vi "Save to File.vi"(8 "error in (no error)":errorcluster, 10 "Single Channel?":bool, 11 "File Control":T1) -> (0 "error out":errorcluster)   [LabVIEW 2017]
uses:
  Controls/File Controls.ctl
  <vilib>/Waveform/WDTFileIO.llb/Read Waveform from File.vi
  <vilib>/Utility/file.llb/Write Delimited Spreadsheet (DBL).vi
panel:
  out "Dev2 + Trigger Signals":dbl[][](array[numeric])
  out "Dev1 Signals":dbl[][](array[numeric])
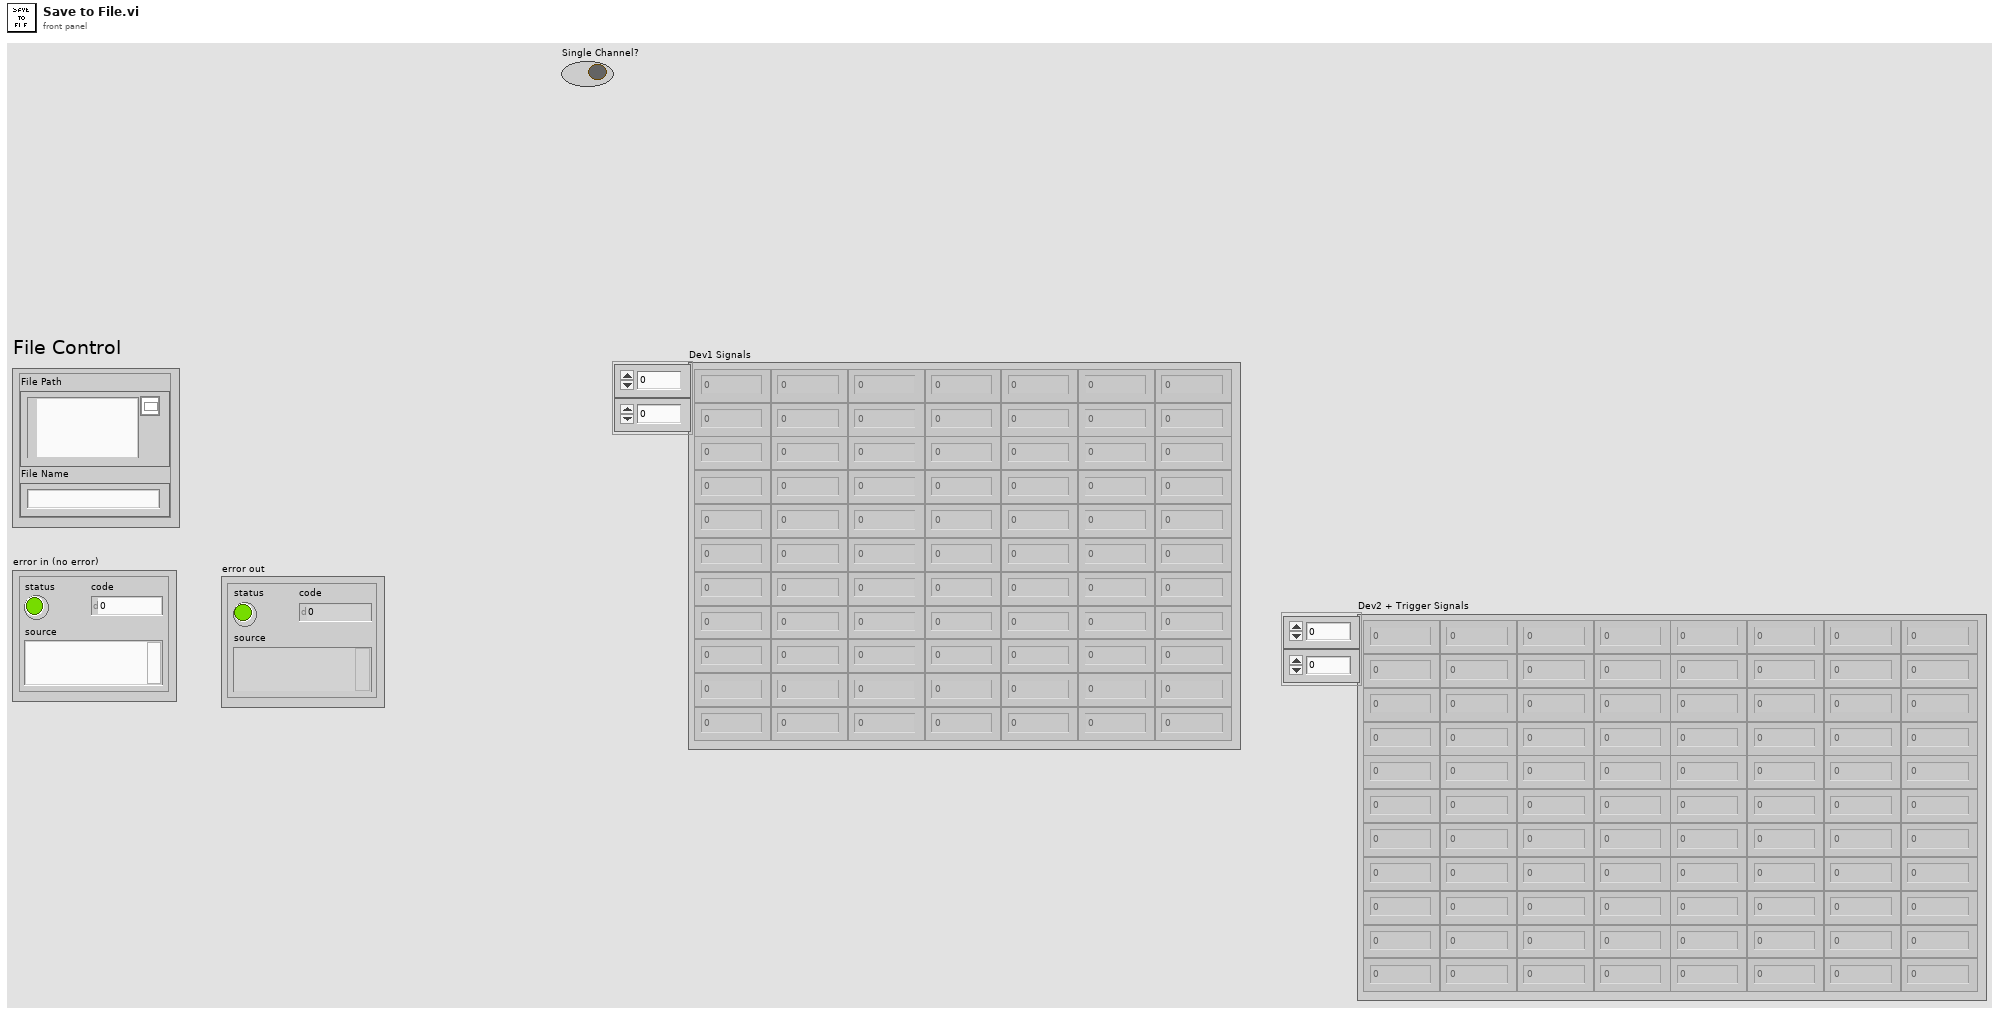
[diagram p1: front panel]
types:
  T1 = typedef "File Controls.ctl" = cluster{"File Path":path, "File Name":string}
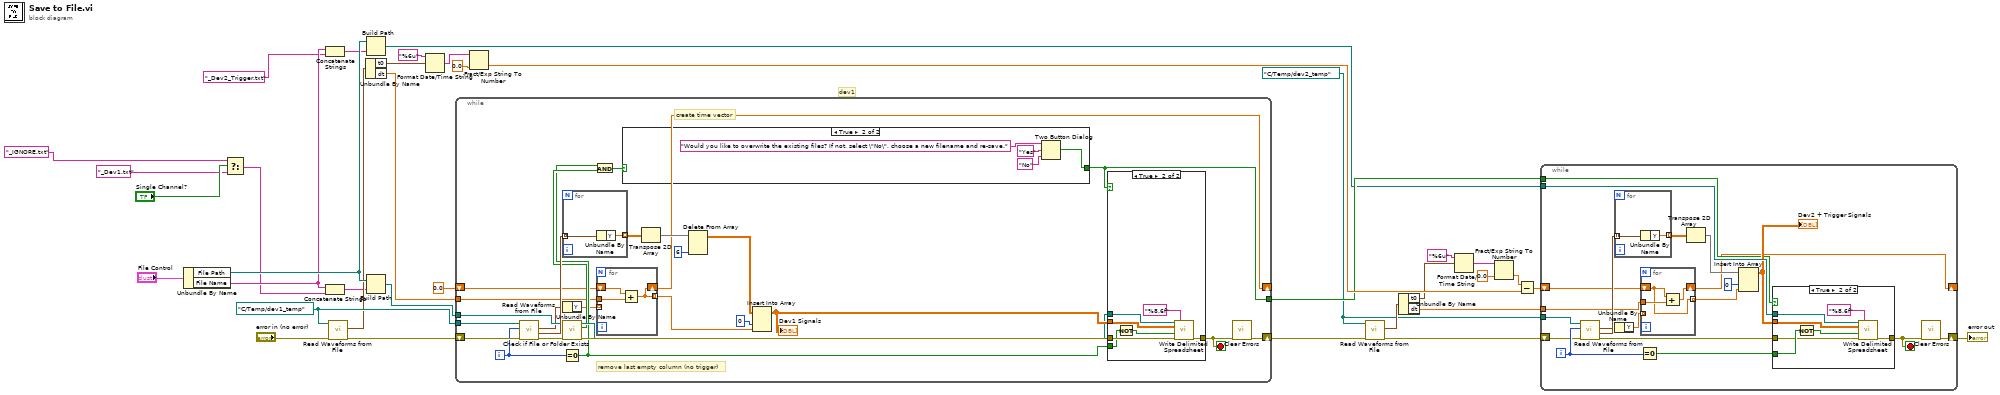
[diagram p0: block diagram]
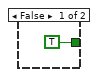
[diagram p3: hidden frame]
diagram:
  w30 = path "C:/Temp/dev1_temp" ("file path (dialog if empty)")
  w13 = path "C:/Temp/dev2_temp" ("file path (dialog if empty)")
  # "dev1"
  n1 = Unbundle By Name("File Control") -> ("File Path"=w35:path, "File Name"=w34:string)
  n2 = Select(t="_IGNORE.txt" ("string"), s="Single Channel?", f="_Dev1.txt" ("string")) -> (s? t:f=w5:string)
  n3 = Concatenate Strings(w34, "_Dev2_Trigger.txt" ("string")) -> (w33:string)
  n4 = Concatenate Strings(w34, w5) -> (w12:string)
  n5 = call-poly <vilib>:"Read Waveforms from File.vi"("error in (no error)"="error in (no error)", "file path (dialog if empty)"=w30) -> ("error out"=w8:errorcluster, "first waveform in record"=w21:waveform(dbl))  [unwired: 4 in, 2 out]
  n6 = Unbundle By Name(w21) -> ("t0"=w20:timestamp, "dt"=w17:dbl)
  n7 = Build Path(base path=w35, name or relative path=w33) -> (appended path=w10:path)
  n8 = Build Path(base path=w35, name or relative path=w12) -> (appended path=w11:path)
  n9 = Format Date/Time String(time format string (%c)="%6u", seconds (now)=w20) -> (date/time string=w26:string)  [unwired: 1 in]
  n10 = while {
    tunnel: w30 -> [w62]
    shift-right: [w51] -> w7
    shift-left: w8 -> [w61]
    shift-right: [w38] -> _
    shift-left: 0.0 -> [w40]
    tunnel: w17 -> [w41]
    tunnel: [w46] -> w16
    tunnel: w11 -> [w44]
    i -> [w48]
    stop <- w50 stop-if-true
    # "create time vector"
    # "remove last empty column (no trigger)"
    n11 = call-poly <vilib>:"Read Waveforms from File.vi"("error in (no error)"=w61, "offset (records:0)"=w48, "file path (dialog if empty)"=w62) -> ("error out"=w45:errorcluster, "all waveforms in record"=w60:waveform(dbl)[], "first waveform in record"=w43:waveform(dbl))  [unwired: 3 in, 1 out]
    n12 = for {
      tunnel: w60 -> [w80] mode=indexing
      tunnel: [w79] -> w59 mode=indexing
      n13 = Unbundle By Name(w80) -> ("Y"=w79:dbl[])
    }
    n14 = Unbundle By Name(w43) -> ("Y"=w42:dbl[])
    n15 = call <vilib>:"Check if File or Folder Exists.vi"("error in (no error)"=w45, "path"=w44) -> ("error out"=w54:errorcluster, "file or folder exists?"=w52:bool, "dup path"=w53:path)  [unwired: 7 in]
    n16 = Equal To 0?(x=w48) -> (x = 0?=w47:bool)
    n17 = And(x=w47, y=w52) -> (x .and. y?=w49:bool)
    n18 = for {
      tunnel: w42 -> [_] mode=indexing
      tunnel: w41 -> [w65]
      shift-right: [w63] -> w38
      shift-left: w40 -> [w64]
      tunnel: [w63] -> w39 mode=indexing
      n19 = Add(x=w64, y=w65) -> (x+y=w63:dbl)
    }
    n20 = case shown="True" w49 {
      tunnel: [TRUE ("T button?") w70] -> w46
      frame False {
      }
      frame True {
        n21 = Two Button Dialog(message="Would you like to overwrite the existing files? If not, select \"No\", choose a new filename and re-save.", 1:"No" ("F button name (\"Cancel\")"), 2:"Yes" ("T button name (\"OK\")")) -> (T button?=w70:bool)
      }
    }
    n22 = Transpose 2D Array(2D array=w59) -> (transposed array=w58:dbl[][])
    n23 = Delete From Array(array=w58, index (col)=6 ("disabled index (col)")) -> (array with subset deleted=w57:dbl[][])  [unwired: 2 in, 1 out]
    n24 = Insert Into Array(array=w57, index (col)=0 ("disabled index (col)"), new element=w39) -> (w55:dbl[][])  [unwired: 1 in]
    "Dev1 Signals" <- w55
    n25 = case shown="True" w46 {
      tunnel: [w71 w72] -> w50
      tunnel: w55 -> [_ w78]
      tunnel: w53 -> [_ w77]
      tunnel: w54 -> [w71 w76]
      tunnel: w47 -> [_ w74]
      frame False {
      }
      frame True {
        n26 = Not(x=w74) -> (.not. x?=w73:bool)
        n27 = call-poly <vilib>:"Write Delimited Spreadsheet.vi"("file path (dialog if empty)"=w77, "format (%.3f)"="%8.6f", "2D data"=w78, "append to file? (new file:F)"=w73, "error in (no error)"=w76) -> ("error out"=w72:errorcluster)  [unwired: 9 in, 1 out]
      }
    }
    n28 = call <vilib>:"Clear Errors.vi"("error in (no error)"=w50) -> ("error out"=w51:errorcluster)  [unwired: 5 in, 1 out]
  }
  n29 = Fract/Exp String To Number(string=w26, default (0 dbl)=0.0 ("default (0 DBL)")) -> (number=w28:dbl)  [unwired: 2 in, 1 out]
  n30 = call-poly <vilib>:"Read Waveforms from File.vi"("error in (no error)"=w7, "file path (dialog if empty)"=w13) -> ("error out"=w6:errorcluster, "first waveform in record"=w18:waveform(dbl))  [unwired: 4 in, 2 out]
  n31 = Unbundle By Name(w18) -> ("t0"=w19:timestamp, "dt"=w9:dbl)
  n32 = Format Date/Time String(time format string (%c)="%6u", seconds (now)=w19) -> (date/time string=w23:string)  [unwired: 1 in]
  n33 = Fract/Exp String To Number(string=w23, default (0 dbl)=0.0 ("default (0 DBL)")) -> (number=w29:dbl)  [unwired: 2 in, 1 out]
  n34 = Subtract(x=w29, y=w28) -> (x-y=w14:dbl)
  n35 = while {
    tunnel: w13 -> [w100]
    tunnel: w10 -> [w95]
    shift-right: [w93] -> w15
    shift-left: w6 -> [w88]
    shift-right: [w82] -> _
    shift-left: w14 -> [w83]
    tunnel: w9 -> [w84]
    tunnel: w16 -> [w89]
    i -> [w91]
    stop <- w92 stop-if-true
    n36 = call-poly <vilib>:"Read Waveforms from File.vi"("error in (no error)"=w88, "offset (records:0)"=w91, "file path (dialog if empty)"=w100) -> ("error out"=w87:errorcluster, "all waveforms in record"=w98:waveform(dbl)[], "first waveform in record"=w86:waveform(dbl))  [unwired: 3 in, 1 out]
    n37 = for {
      tunnel: w98 -> [w113] mode=indexing
      tunnel: [w112] -> w97 mode=indexing
      n38 = Unbundle By Name(w113) -> ("Y"=w112:dbl[])
    }
    n39 = Unbundle By Name(w86) -> ("Y"=w85:dbl[])
    n40 = Equal To 0?(x=w91) -> (x = 0?=w90:bool)
    n41 = for {
      tunnel: w85 -> [_] mode=indexing
      tunnel: w84 -> [w103]
      shift-right: [w102] -> w82
      shift-left: w83 -> [w101]
      tunnel: [w101] -> w81 mode=indexing
      n42 = Add(x=w101, y=w103) -> (x+y=w102:dbl)
    }
    n43 = Transpose 2D Array(2D array=w97) -> (transposed array=w96:dbl[][])
    n44 = Insert Into Array(array=w96, index (col)=0 ("disabled index (col)"), new element=w81) -> (w94:dbl[][])  [unwired: 1 in]
    "Dev2 + Trigger Signals" <- w94
    n45 = case shown="True" w89 {
      tunnel: [w104 w111] -> w92
      tunnel: w95 -> [_ w110]
      tunnel: w94 -> [_ w109]
      tunnel: w87 -> [w104 w105]
      tunnel: w90 -> [_ w107]
      frame False {
      }
      frame True {
        n46 = Not(x=w107) -> (.not. x?=w106:bool)
        n47 = call-poly <vilib>:"Write Delimited Spreadsheet.vi"("file path (dialog if empty)"=w110, "format (%.3f)"="%8.6f", "2D data"=w109, "append to file? (new file:F)"=w106, "error in (no error)"=w105) -> ("error out"=w111:errorcluster)  [unwired: 9 in, 1 out]
      }
    }
    n48 = call <vilib>:"Clear Errors.vi"("error in (no error)"=w92) -> ("error out"=w93:errorcluster)  [unwired: 5 in, 1 out]
  }
  "error out" <- w15
